vi "KV_CurHead_Addr_Set.vi"(9 "设置的新地址":u8=1 min=1 max=10 step=1, 10 "原来地址":u8=1 min=1 max=10 step=1, 11 "MyIndex":u8) -> (3 "OK?":bool)   [LabVIEW 2015]
uses:
  <vilib>/Instr/_visa.llb/VISA Configure Serial Port (Instr).vi
panel:
  out "字符串":string
  out "InPut +CRC":string
  out "VISA":refnum<visa-resource-name> caption="VISA资源名称输出"
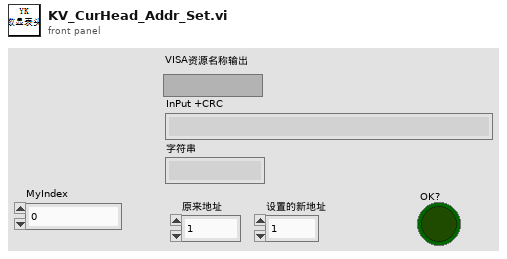
[diagram p1: front panel]
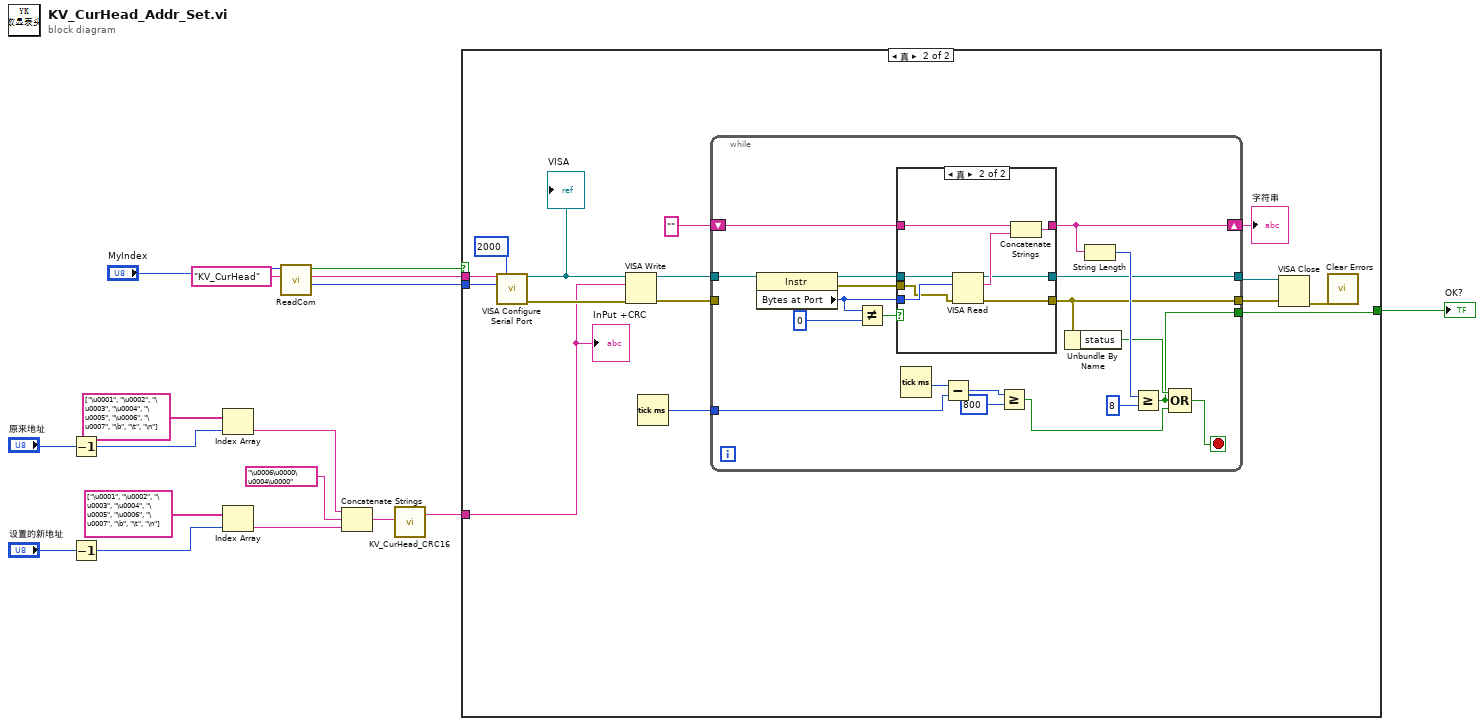
[diagram p0: block diagram]
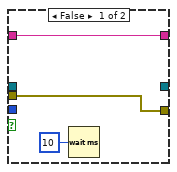
[diagram p3: hidden frame]
diagram:
  n1 = Decrement(x="原来地址") -> (x-1=w8:u8)
  n2 = Decrement(x="设置的新地址") -> (x-1=w7:u8)
  n3 = Index Array(array=string[] ["\u0001", "\u0002", "\u0003", "\u0004", "\u0005", "\u0006", "\u0007", "\b", "\t", "\n"], index=w8) -> (element=w13:string)
  n4 = Index Array(array=string[] ["\u0001", "\u0002", "\u0003", "\u0004", "\u0005", "\u0006", "\u0007", "\b", "\t", "\n"], index=w7) -> (element=w11:string)
  n5 = call "ReadCom.vi"("仪器名称"="KV_CurHead", "MyIndex"="MyIndex") -> ("Baudrate"=w1:i32, "COM"=w2:string, "OK?"=w3:bool)  [unwired: 7 in]
  n6 = Concatenate Strings(w13, "\u0006\u0000\u0004\u0000" ("字符串"), w11) -> (w10:string)
  n7 = call "KV_CurHead_CRC16.vi"("input String"=w10) -> ("InPut +CRC"=w9:string)  [unwired: 1 out]
  n8 = case shown="真" w3 {
    tunnel: w9 -> [_ w26]
    tunnel: [_ w25] -> w6
    tunnel: w2 -> [_ w24]
    tunnel: w1 -> [_ w19]
    frame False {
    }
    frame True {
      n9 = call-poly "VISA Configure Serial Port"("VISA resource name"=w24, "timeout (10sec)"=u32 2000, "baud rate (9600)"=w19) -> ("VISA resource name out"=w32:refnum<visa-resource-name>, "error out"=w31:errorcluster)  [unwired: 11 in]
      "VISA" <- w32
      n10 = VISA Write(VISA resource name=w32, write buffer=w26, error in (no error)=w31) -> (VISA resource name out=w29:refnum<visa-resource-name>, error out=w30:errorcluster)  [unwired: 1 out]
      n11 = Tick Count (ms)() -> (millisecond timer value=w27:u32)
      n12 = while {
        tunnel: w30 -> [_]
        tunnel: w29 -> [w52]
        shift-right: [w45] -> w18
        shift-left: "" -> [w46]
        tunnel: w27 -> [w39]
        tunnel: [w35] -> w25
        tunnel: [w34] -> w22
        tunnel: [w33] -> w21
        stop <- w42 stop-if-true
        n13 = property class="Instr"(reference=w52) -> (reference out=w49:refnum<visa-resource-name>, error out=w47:errorcluster, "Bytes at Port"=w48:u32)  [unwired: 1 in]
        n14 = Not Equal?(x=w48, y=u32 0) -> (x != y?=w50:bool)
        n15 = case shown="真" w50 {
          tunnel: w49 -> [_ w63]
          tunnel: w48 -> [_ w62]
          tunnel: w47 -> [w53 w61]
          tunnel: w46 -> [w54 w60]
          tunnel: [w54 w58] -> w45
          tunnel: [w53 w57] -> w33
          tunnel: [_ w56] -> w34
          frame False {
            n16 = Wait (ms)(milliseconds to wait=u32 10 ("等待时间（毫秒）")) -> ()  [unwired: 1 out]
          }
          frame True {
            n17 = VISA Read(VISA resource name=w63, byte count=w62, error in (no error)=w61) -> (VISA resource name out=w56:refnum<visa-resource-name>, read buffer=w59:string, error out=w57:errorcluster)  [unwired: 1 out]
            n18 = Concatenate Strings(w60, w59) -> (w58:string)
          }
        }
        n19 = Tick Count (ms)() -> (millisecond timer value=w40:u32)
        n20 = Subtract(x=w40, y=w39) -> (x-y=w38:u32)
        n21 = Greater Or Equal?(x=w38, y=u32 800) -> (x >= y?=w36:bool)
        n22 = Unbundle By Name(w33) -> ("status"=w41:bool)
        n23 = String Length(string=w45) -> (length=w44:i32)
        n24 = Greater Or Equal?(x=w44, y=8) -> (x >= y?=w35:bool)
        n25 = Compound Arithmetic op=OR ("复合运算")(w41, w35, w36) -> (w42:bool)
      }
      "字符串" <- w18
      n26 = VISA Close(VISA resource name=w22, error in (no error)=w21) -> (error out=w20:errorcluster)
      n27 = call <vilib>:"Clear Errors.vi"("error in (no error)"=w20) -> ()  [unwired: 5 in, 2 out]
      "InPut +CRC" <- w26
    }
  }
  "OK?" <- w6
